vi "HSMS Initialize.vi"(8 "error in (no error)":errorcluster, 11 "Role":T1) -> (0 "error out":errorcluster, 3 "HSMS Class out":refnum<class "HSMS Class.lvclass">)   [LabVIEW 2020, in "SECS Communication.lvlib" / "HSMS Class.lvclass"]
uses:
  HSMS Class.lvclass
  Role.ctl
  Command Data.ctl
  SECS-II Class/SECS-II Class.lvclass
  HSMS State Data.ctl
  HSMS State.ctl
  Notifier Data.ctl
  Notifier Type.ctl
  HSMS Class.lvclass/HSMS Class.ctl
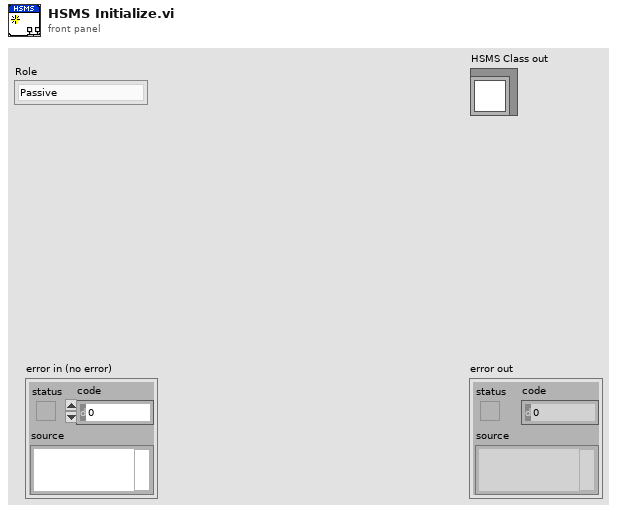
[diagram p1: front panel]
types:
  T1 = typedef "SECS Communication.lvlib/HSMS Class.lvclass/Role.ctl" = enum16{"Passive", "Active"}
  T2 = typedef "SECS Communication.lvlib/HSMS Class.lvclass/Notifier Data.ctl" = cluster{"Notifier Type":T3, "Data":variant, "Time":timestamp}
  T3 = typedef "SECS Communication.lvlib/HSMS Class.lvclass/Notifier Type.ctl" = enum16{"TCPIP Connect", "TCPIP Disconnect", "Receive Message", "Send Message", "T3 Timeout", "T6 Timeout", "T7 Timeout", "Error", "Stop"}
  T4 = typedef "SECS Communication.lvlib/HSMS Class.lvclass/HSMS State Data.ctl" = cluster{"HSMS State":T5, "T3(Reply Timeout)":i32, "T5(Separation Timeout)":i32, "T6(Control Timeout)":i32, "T7(Not Selected Timeout)":i32, "T8(Inter-Character Timeout)":i32, "Session ID":u16, "Alive Notifier":refnum<notifier>, "Log Path":path, "Listener Refnum":refnum<k5>}
  T5 = typedef "SECS Communication.lvlib/HSMS Class.lvclass/HSMS State.ctl" = enum16{"[TCP/IP]Not Connect", "[HSMS]Not Selected", "[HSMS]Selected", "Stop"}
  T6 = typedef "SECS Communication.lvlib/HSMS Class.lvclass/Command Data.ctl" = cluster{"SECS-II Class":refnum<class "SECS-II Class.lvclass">, "Reply Notifier":refnum<notifier>}
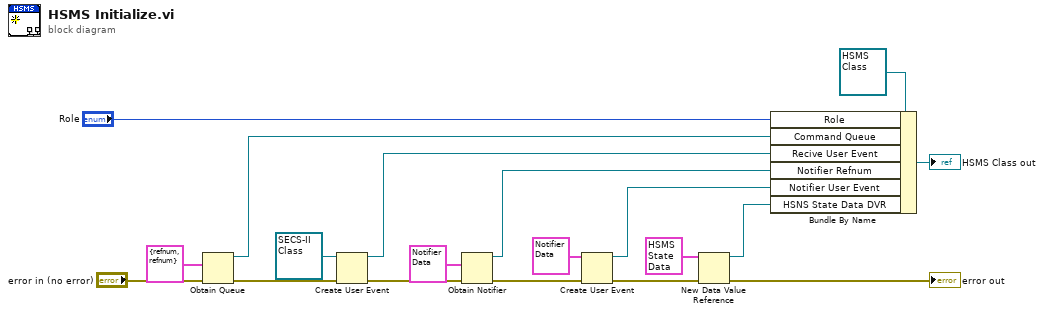
[diagram p0: block diagram]
diagram:
  n1 = Obtain Queue(element data type=T6 {"SECS-II Class"=refnum, "Reply Notifier"=refnum} ("Command Data"), error in (no error)="error in (no error)") -> (queue out=w14:refnum<queue>, error out=w19:errorcluster)  [unwired: 3 in, 1 out]
  n2 = Create User Event(user event datatype=refnum<class "SECS-II Class.lvclass"> refnum ("SECS Communication.lvlib:SECS-II Class.lvclass"), error in=w19) -> (user event=w17:refnum<user-event>, error out=w18:errorcluster)
  n3 = Obtain Notifier(notification data type=T2 {"Notifier Type"=enum."Send Message", "Data"=variant, "Time"=timestamp(0 s since 1904-01-01)} ("Notifier Data"), error in (no error)=w18) -> (notifier out=w11:refnum<notifier>, error out=w4:errorcluster)  [unwired: 2 in, 1 out]
  n4 = Create User Event(user event datatype=T2 {"Notifier Type"=enum."Send Message", "Data"=variant, "Time"=timestamp(0 s since 1904-01-01)} ("Notifier Data"), error in=w4) -> (user event=w3:refnum<user-event>, error out=w2:errorcluster)
  n5 = New Data Value Reference(data value=T4 {"HSMS State"=enum."Stop", "T3(Reply Timeout)"=45000, "T5(Separation Timeout)"=10000, "T6(Control Timeout)"=5000, "T7(Not Selected Timeout)"=1000, "T8(Inter-Character Timeout)"=5000, "Session ID"=0, "Alive Notifier"=refnum, "Log Path"=path "D:/SECS", "Listener Refnum"=refnum} ("HSMS State Data"), error in=w2) -> (data value reference=w5:refnum<data-value>, error out=→"error out":errorcluster)
  n6 = Bundle By Name(cluster=refnum<class "HSMS Class.lvclass"> refnum ("HSMS Class in"), "Role"="Role", "Command Queue"=w14, "Recive User Event"=w17, "Notifier Refnum"=w11, "Notifier User Event"=w3, "HSNS State Data DVR"=w5) -> (→"HSMS Class out":refnum<class "HSMS Class.lvclass">)
